vi "XImc example calb.vi"() -> ()   [LabVIEW 2012]
uses:
  libximc.lvlib
panel:
  in  "error in (no error)":errorcluster
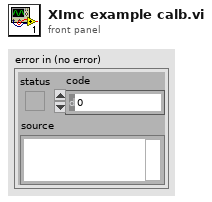
[diagram p1: front panel]
types:
  T1 = cluster{"NomVoltage":u32, "NomCurrent":u32, "NomSpeed":u32, "uNomSpeed":u32, "EngineFlags":u32, "Antiplay":i32, "MicrostepMode":u32, "StepsPerRev":u32}
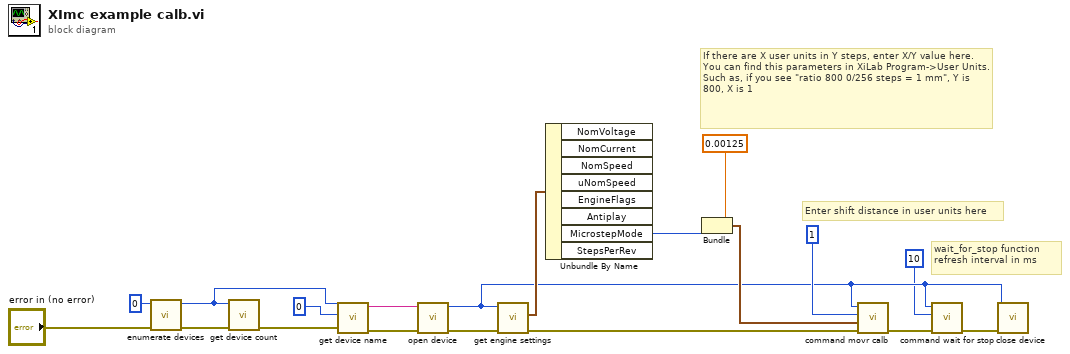
[diagram p0: block diagram]
diagram:
  # "wait_for_stop function refresh interval in ms"
  # "Enter shift distance in user units here"
  # "If there are X user units in Y steps, enter X/Y value here.\nYou can find this parameters in XiLab Program->User Units.\nSuch as, if you see \"ratio 800 0/256 steps = 1 mm\", Y is 800, X is 1"
  n1 = call "enumerate devices.vi"("error in (no error)"="error in (no error)", "enumerate_flags"=0 ("probe_devices")) -> ("error out"=w17:errorcluster, "function return"=w15:u64)  [unwired: 8 in]
  n2 = call "get device count.vi"("error in (no error)"=w17, "device_enumeration"=w15) -> ("error out"=w16:errorcluster)  [unwired: 8 in, 1 out]
  n3 = call "get device name.vi"("error in (no error)"=w16, "device_index"=0 ("probe_devices"), "device_enumeration"=w15) -> ("error out"=w12:errorcluster, "function return"=w13:string)  [unwired: 7 in]
  n4 = call "open device.vi"("error in (no error)"=w12, "name"=w13) -> ("error out"=w10:errorcluster, "function return"=w3:i32)  [unwired: 8 in]
  n5 = call "get engine settings.vi"("error in (no error)"=w10, "id"=w3) -> ("error out"=w5:errorcluster, "engine_settings out"=w9:T1)  [unwired: 7 in, 1 out]
  n6 = Unbundle By Name(w9) -> ("MicrostepMode"=w8:u32)  [unwired: 7 out]
  n7 = Bundle(0.00125, "MicrostepMode"=w8) -> (w6:cluster{dbl, "MicrostepMode":u32})  [unwired: 1 in]
  n8 = call "command movr calb.vi"("error in (no error)"=w5, "calibration"=w6, "DeltaPosition"=1 ("probe_devices"), "id"=w3) -> ("error out"=w4:errorcluster)  [unwired: 6 in, 1 out]
  n9 = call "command wait for stop.vi"("error in (no error)"=w4, "refresh_interval_ms"=10 ("probe_devices"), "id"=w3) -> ("error out"=w1:errorcluster)  [unwired: 7 in, 1 out]
  n10 = call "close device.vi"("error in (no error)"=w1, "id"=w3) -> ()  [unwired: 7 in, 3 out]
